vi "Read.vi"(8 "error in (no error)":errorcluster, 11 "Boolean in":refnum<class "Const_Bool_1D.lvclass">) -> (0 "error out":errorcluster, 2 "Array":bool[](array[boolean]), 3 "Boolean out":refnum<class "Const_Bool_1D.lvclass">)   [LabVIEW 2021, in "Const_Bool_1D.lvclass"]
uses:
  Const_Bool_1D.lvclass
  Const_Bool_1D.lvclass/Const_Bool_1D.ctl
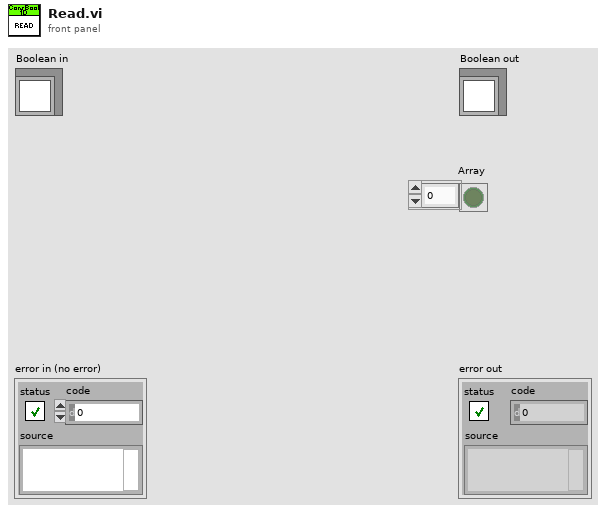
[diagram p1: front panel]
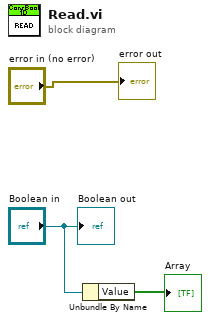
[diagram p0: block diagram]
diagram:
  n1 = Unbundle By Name("Boolean in") -> ("Value"=→"Array":bool[])
  "error out" <- "error in (no error)"
  "Boolean out" <- "Boolean in"
